vi "Spreadsheet Storage.vi"() -> ()   [LabVIEW 2017]
uses:
  <vilib>/Utility/file.llb/Write Delimited Spreadsheet (DBL).vi
panel:
  in  "Waveform Parameters":T1={"Frequency"=50.0, "Amplitude"=5.0, "Shape"=enum."Sine"}
  in  "Digitizing Parameters":T2={"Numbers of Samples"=100, "Sampling Frequency"=1000.0}
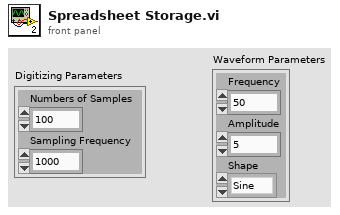
[diagram p1: front panel]
types:
  T1 = cluster{"Frequency":dbl, "Amplitude":dbl, "Shape":enum16{"Sine", "Cosine", "DC Level", "Square", "User-Defined"}}
  T2 = cluster{"Numbers of Samples":i32, "Sampling Frequency":dbl}
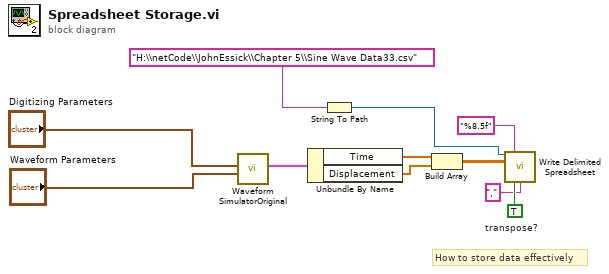
[diagram p0: block diagram]
diagram:
  w8 = TRUE  # transpose?
  # "How to store data effectively"
  n1 = call "Waveform SimulatorOriginal.vi"("Waveform Parameters"="Waveform Parameters", "Digitizing Parameters"="Digitizing Parameters") -> ("Waveform Output"=w9:cluster{"Time":dbl[], "Displacement":dbl[]})  [unwired: 9 in]
  n2 = Unbundle By Name(w9) -> ("Time"=w7:dbl[], "Displacement"=w6:dbl[])
  n3 = String To Path(string="H:\\netCode\\JohnEssick\\Chapter 5\\Sine Wave Data33.csv" ("format (%.3f)")) -> (path=w4:path)
  n4 = Build Array(w7, w6) -> (w2:dbl[][])
  n5 = call-poly <vilib>:"Write Delimited Spreadsheet.vi"("file path (dialog if empty)"=w4, "format (%.3f)"="%8.5f", "2D data"=w2, "transpose? (no:F)"=w8, "delimiter (\\t)"="," ("delimiter (\\t)")) -> ()  [unwired: 9 in, 2 out]
